vi "proyecto.vi"() -> ()   [LabVIEW 2020]
panel:
  out "ALARMA":bool
  out "BOMBA 3":bool
  in  "MARCHA 3":bool
  in  "PARO 3":bool
  out "BOMBA 2":bool
  in  "MARCHA 2":bool
  in  "PARO 2":bool
  out "BOMBA 1":bool
  in  "MARCHA 1":bool
  in  "PARO 1":bool
  in  "SOLO PARA EMERGENCIA":bool
  in  "Selector de modo":bool
  out "MODO":string
  out "Medidor Presion":dbl
  in  "Boolean 3":bool
  in  "Boolean 2":bool
  in  "Boolean":bool
  in  "Presion":dbl(slide) scale=0.0..5.0
  in  "stop":bool
  # "Manual"
  # "Automático"
  # "OFF                ON"
  # "OFF                ON"
  # "OFF                ON"
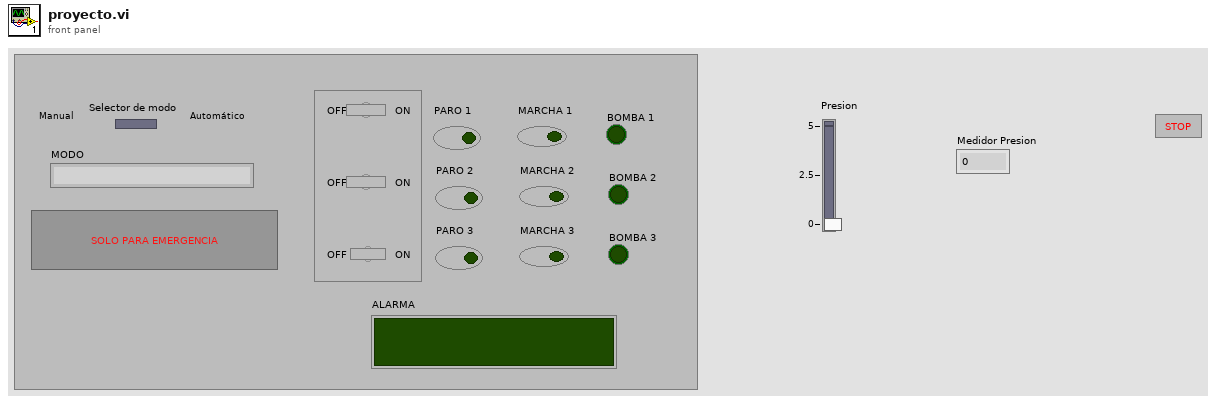
[diagram p1: front panel]
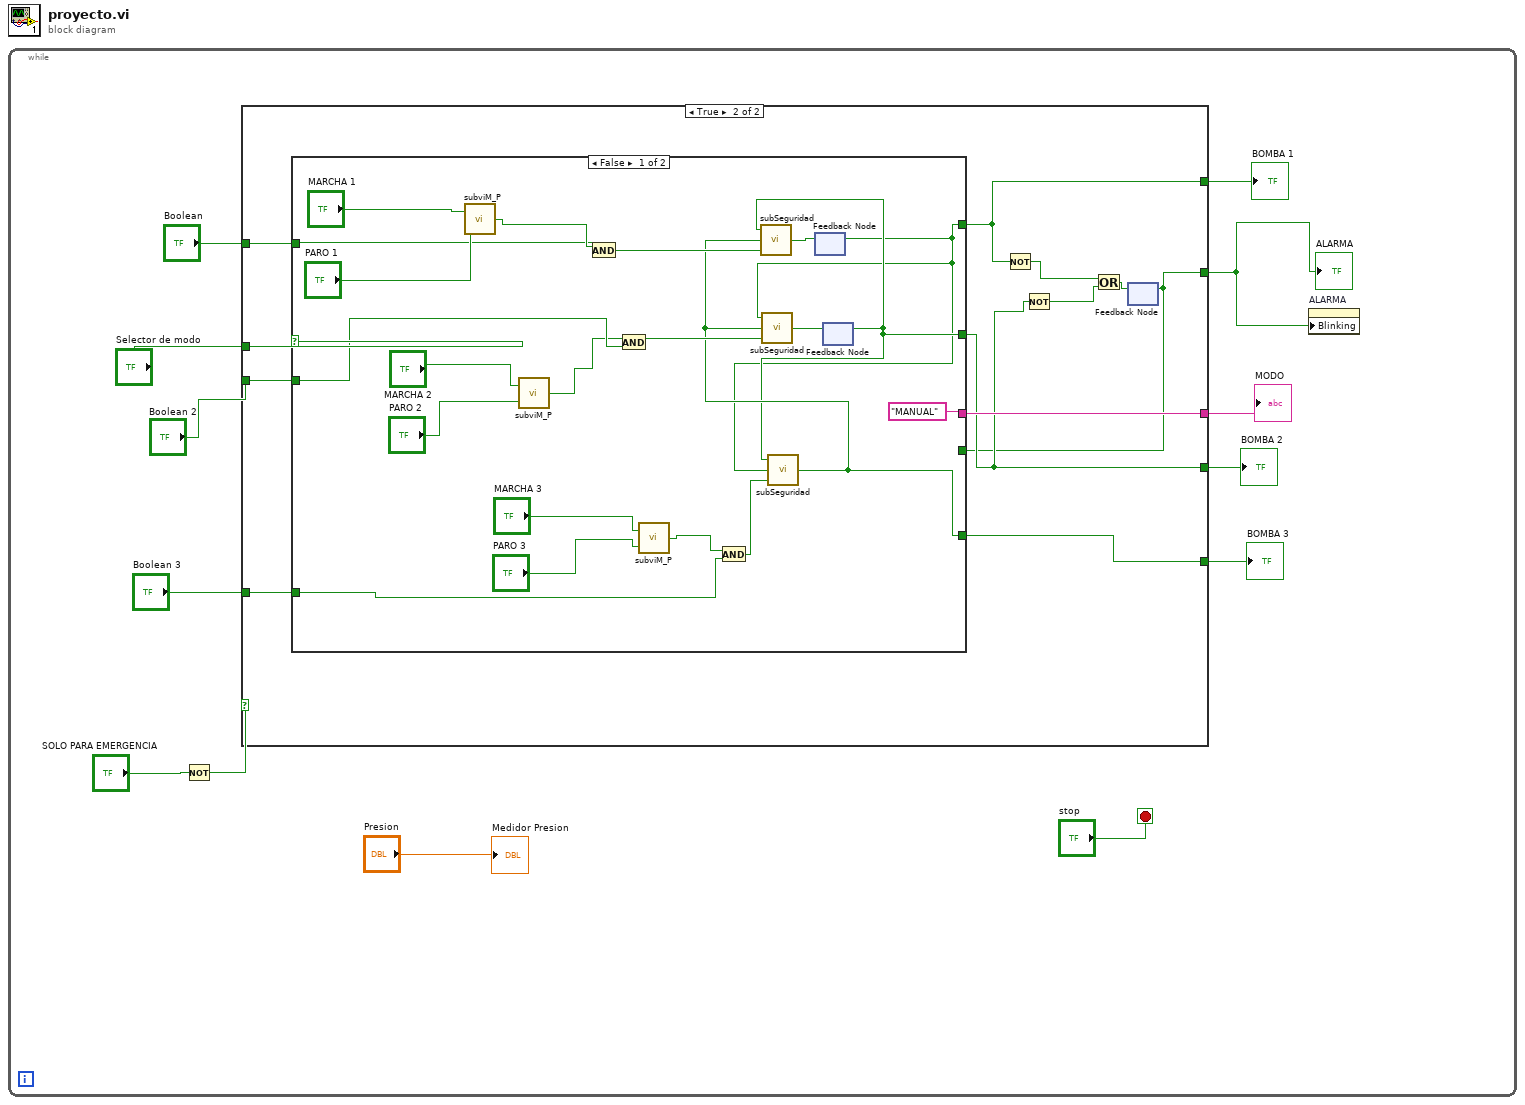
[diagram p0: block diagram]
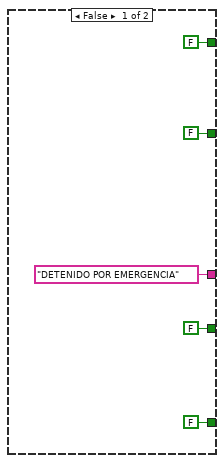
[diagram p2: hidden frame]
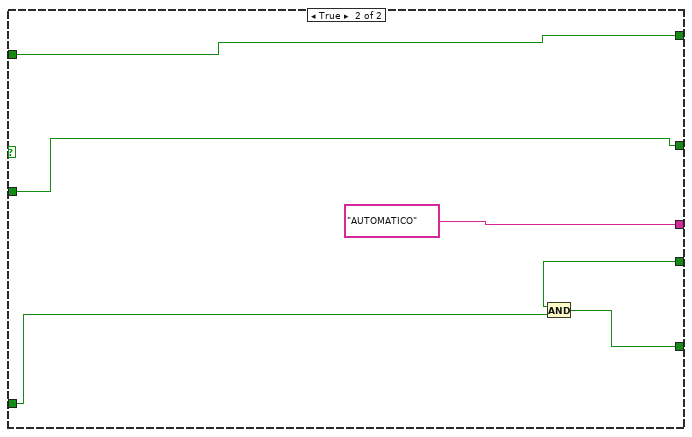
[diagram p3: hidden frame]
diagram:
  n1 = while {
    stop <- "stop" stop-if-true
    n2 = Not(x="SOLO PARA EMERGENCIA") -> (.not. x?=w3:bool)
    n3 = case shown="True" w3 {
      tunnel: ["DETENIDO POR EMERGENCIA" w30] -> w13
      tunnel: "Selector de modo" -> [_ w29]
      tunnel: [FALSE (".not. (x .and. y)?") w28] -> w10
      tunnel: "Boolean" -> [_ w27]
      tunnel: "Boolean 2" -> [_ w26]
      tunnel: "Boolean 3" -> [_ w25]
      tunnel: [FALSE ("Boolean") w24] -> w6
      tunnel: [FALSE ("Boolean 2") w22] -> w5
      tunnel: [FALSE w19] -> w1
      frame False {
      }
      frame True {
        n4 = feedback #1() -> (w19:bool)  [unwired: 1 in]
        n5 = case shown="False" w29 {
          tunnel: ["MANUAL" "AUTOMATICO"] -> w30
          tunnel: [w34 w54] -> w28
          tunnel: [w33 w56] -> w22
          tunnel: [w31 w55] -> w24
          tunnel: w27 -> [w43 w55]
          tunnel: w26 -> [w42 w56]
          tunnel: w25 -> [w40 w52]
          tunnel: w19 -> [_ w53]
          frame False {
            n6 = call "subviM_P.vi"("PARO in"="PARO 1", "MARCHA in"="MARCHA 1") -> ("Boolean"=w44:bool)
            n7 = call "subviM_P.vi"("PARO in"="PARO 2", "MARCHA in"="MARCHA 2") -> ("Boolean"=w41:bool)
            n8 = And(x=w44, y=w43) -> (x .and. y?=w38:bool)
            n9 = And(x=w41, y=w42) -> (x .and. y?=w37:bool)
            n10 = call "subviM_P.vi"("PARO in"="PARO 3", "MARCHA in"="MARCHA 3") -> ("Boolean"=w39:bool)
            n11 = And(x=w39, y=w40) -> (x .and. y?=w36:bool)
            n12 = feedback #2() -> (w31:bool)  [unwired: 1 in]
            n13 = feedback #3() -> (w33:bool)  [unwired: 1 in]
            n14 = call "subSeguridad.vi"("z"=w36, "y"=w31, "x"=w33) -> (".not. (x .and. y)?"=w34:bool)
            n15 = call "subSeguridad.vi"("z"=w38, "y"=w34, "x"=w33) -> (".not. (x .and. y)?"=w32:bool)
            n16 = call "subSeguridad.vi"("z"=w37, "y"=w34, "x"=w31) -> (".not. (x .and. y)?"=w35:bool)
            n17 = feedback-in #2(w32) -> ()
            n18 = feedback-in #3(w35) -> ()
          }
          frame True {
            n19 = And(x=w53, y=w52) -> (x .and. y?=w54:bool)
          }
        }
        n20 = Not(x=w24) -> (.not. x?=w23:bool)
        n21 = Not(x=w22) -> (.not. x?=w21:bool)
        n22 = Or(x=w23, y=w21) -> (x .or. y?=w20:bool)
        n23 = feedback-in #1(w20) -> ()
      }
    }
    "MODO" <- w13
    "BOMBA 1" <- w6
    "BOMBA 2" <- w5
    "BOMBA 3" <- w10
    "ALARMA" <- w1
    n24 = property on="ALARMA" class="Bool (strict)"("Blinking"=w1) -> ()  [unwired: 2 in, 2 out]
    "Medidor Presion" <- "Presion"
  }
